vi "ni579x Load Characterization Data (EEPROM).vi"(0 "Register Bus":refnum<class "ni579x Register Bus v1 Host.lvclass">=refnum, 1 "scope":string(combo)="characterization data eeprom", 5 "start address":u32 format="%x", 7 "EEPROM Data Section":T1, 11 "Error In":errorcluster) -> (3 "EEPROM Header":T7 {"Product Code" format="%x"; "Checksum" format="%x"}, 4 "Register Bus (out)":refnum<class "ni579x Register Bus v1 Host.lvclass">, 6 "EEPROM Calibration Header":T6={"Checksum"=0, "Date"=timestamp(0 s since 1904-01-01), "Temperature"=0.0, "Misc. Info"="", "Pointer to Device Data Header"=0, "Number of Reserved Bytes"=28} {"Checksum" format="%x"}, 8 "Device Data Header":T5={"Checksum"=0, "Number of Channels"=0, "Number of Attenuations"=[], "Number of Attenuator Settings"=[], "Number of Gain Settings"=[], "Pointer to Cal Data"=[], "Number of Reserved Bytes"=7, "Number of Frequencies"=[]} {"Checksum" format="%x"}, 10 "Characterization Data":T2[](array[typedef]) {"Frequencies [Hz]" format="%#_6p"}, 15 "Error Out":errorcluster)   [LabVIEW 2013]
doc: "Reads characterization data from the on-device EEPROM and returns headers and an array of characterization data for each channel.\n\n<B>Input Parameters</B>\n\n<B>Register Bus</B> The Register Bus object created by the ni579x Open VI and used as the session handle for the NI-579x Configuration Design Library.\n\n<B>scope</B> The EEPROM to read characterization data from. The only option is \"characterization data eeprom\".\n\n<B>start address</B> The start offset of the data in the EEPROM.\n\n<B>EEPROM Data Section</B> The EEPROM can contain characterization data measured and calculated by the manufacturer (the Factory Data) as well as data measured and calculated by the user (the User Data).\n\n<B>Output Parameters</B>\n\n<B>Register Bus (out)</B> The Register Bus object created by the ni579x Open VI and used as the session handle for the NI-579x Configuration Design Library.\n\n<B>EEPROM Header</B> Header information for the entire EEPROM.\n\n<B>EEPROM Calibration Header</B> Header information describing the calibration sections.\n\n<B>Device Data Header</B> Header information describing the device characterization data sections.\n\n<B>Characterization Data</B> An array of characterization data for each channel.\nFor the 5791,\n the Rx channel is index 0\n the Tx channel is index 1\nFor the 5792,\n the Rx channel is index 0\nFor the 5793,\n the Tx channel is index 1"
uses:
  <instrlib>/ni579x/Register Bus/v1/Host/ni579x Register Bus v1 Host.lvclass
  <instrlib>/ni579x/Config/v1/Shared/Types/EEPROM/ni579x EEPROM Header.ctl
  <instrlib>/ni579x/Config/v1/Shared/Types/EEPROM/ni579x EEPROM Calibration Header.ctl
  <instrlib>/ni579x/Config/v1/Shared/Types/EEPROM/ni579x EEPROM Device Data Header.ctl
  <instrlib>/ni579x/Config/v1/Shared/Types/ni579x Characterization Data.ctl
  <instrlib>/ni579x/Config/v1/Shared/Types/ni579x IQ Imbalance.ctl
  <instrlib>/ni579x/Config/v1/Shared/Types/ni579x Gain to Attenuation Mapping.ctl
  <instrlib>/ni579x/Config/v1/Shared/Types/EEPROM/ni579x EEPROM Data Section.ctl
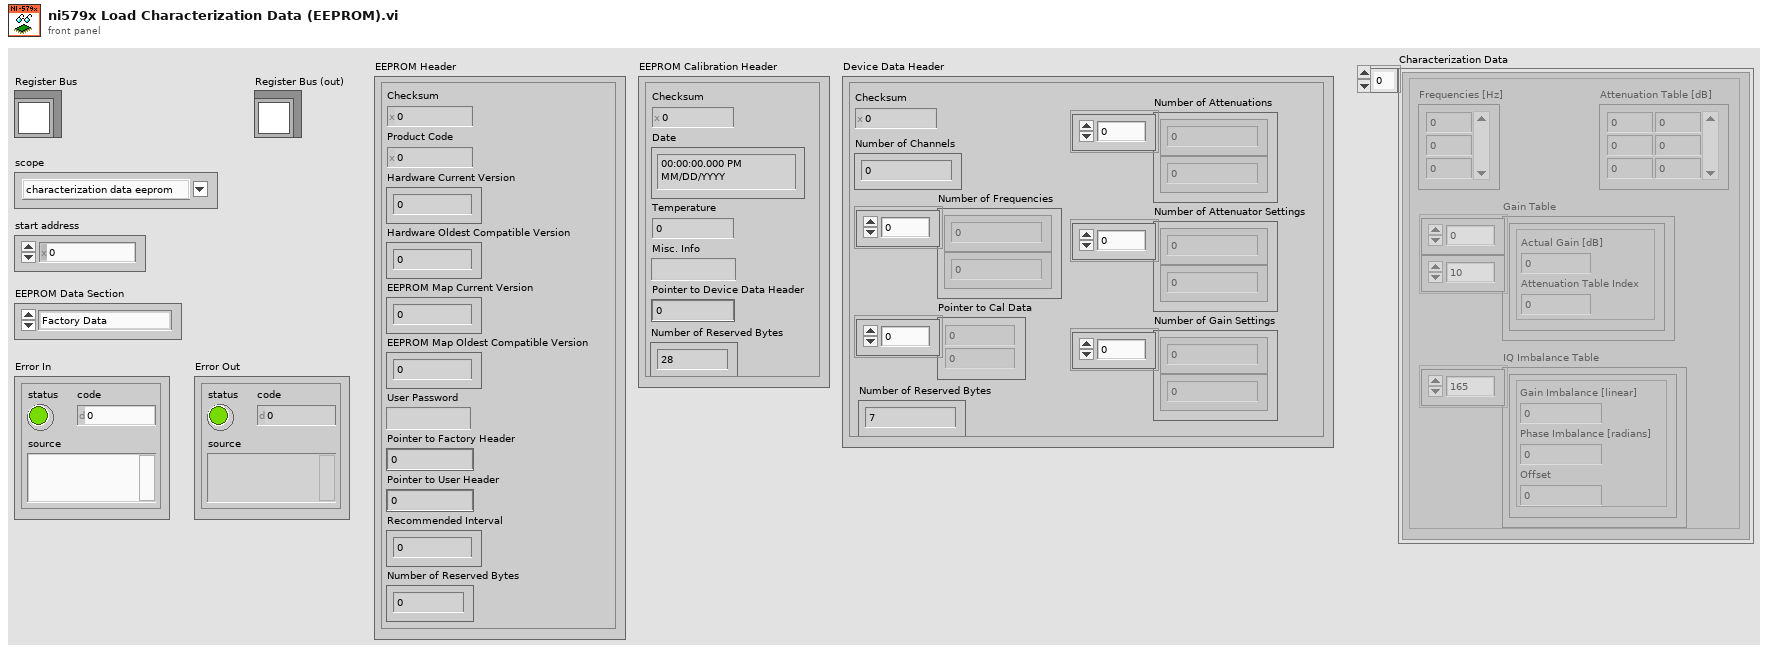
[diagram p1: front panel]
types:
  T1 = typedef "ni579x EEPROM Data Section.ctl" = enum16{"Factory Data", "User Data"}
  T2 = typedef "ni579x Characterization Data.ctl" = cluster{"Attenuation Table [dB]":dbl[][], "Frequencies [Hz]":dbl[], "IQ Imbalance Table":T3[], "Gain Table":T4[][]}
  T3 = typedef "ni579x IQ Imbalance.ctl" = cluster{"Gain Imbalance [linear]":dbl, "Phase Imbalance [radians]":dbl, "Offset":cdb}
  T4 = typedef "ni579x Gain to Attenuation Mapping.ctl" = cluster{"Actual Gain [dB]":dbl, "Attenuation Table Index":i32}
  T5 = typedef "ni579x EEPROM Device Data Header.ctl" = cluster{"Checksum":u32, "Number of Channels":u8, "Number of Attenuations":u16[], "Number of Attenuator Settings":u8[], "Number of Gain Settings":u8[], "Pointer to Cal Data":u32[], "Number of Reserved Bytes":i32, "Number of Frequencies":u16[]}
  T6 = typedef "ni579x EEPROM Calibration Header.ctl" = cluster{"Checksum":u32, "Date":timestamp, "Temperature":sgl, "Misc. Info":string, "Pointer to Device Data Header":u32, "Number of Reserved Bytes":i32}
  T7 = typedef "ni579x EEPROM Header.ctl" = cluster{"Checksum":u32, "Product Code":u16, "Hardware Current Version":u16, "Hardware Oldest Compatible Version":u16, "EEPROM Map Current Version":u16, "EEPROM Map Oldest Compatible Version":u16, "User Password":string, "Pointer to Factory Header":u32, "Pointer to User Header":u32, "Recommended Interval":u16, "Number of Reserved Bytes":i32}
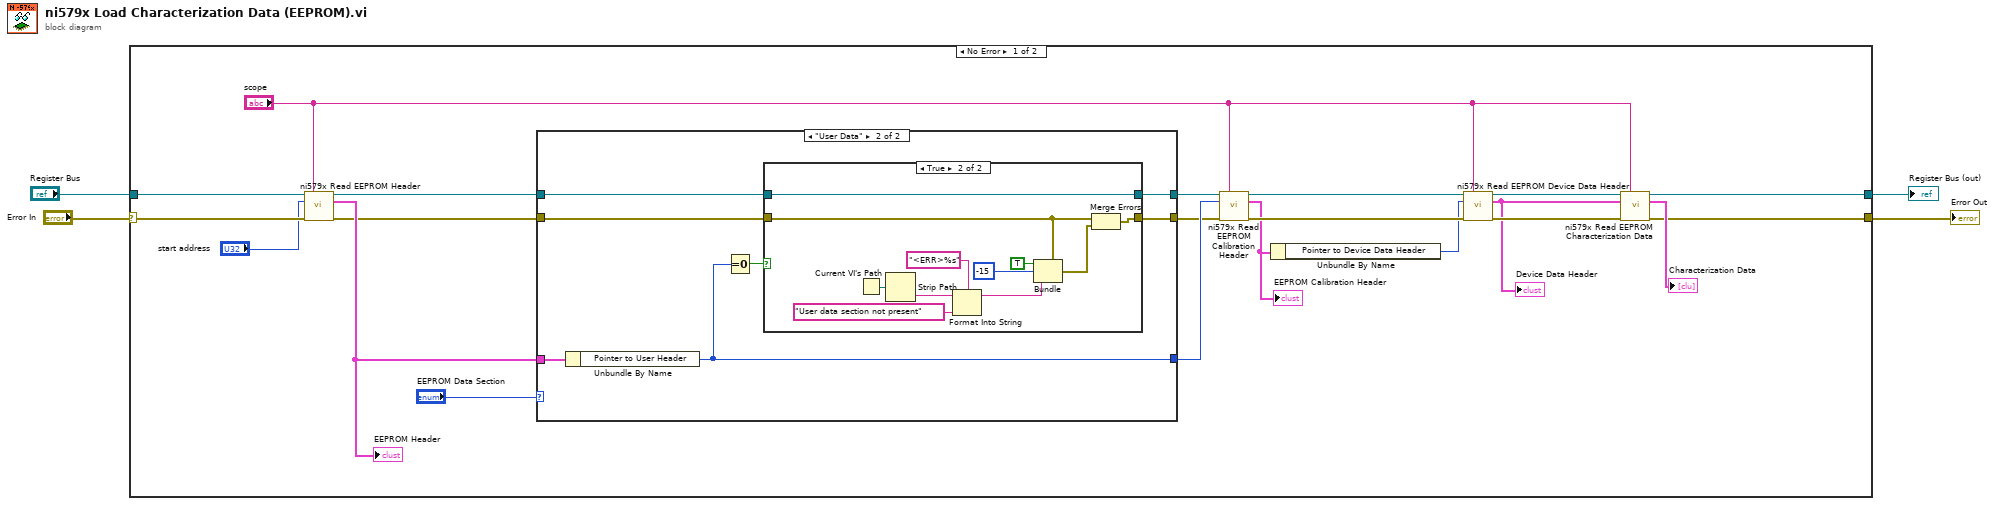
[diagram p0: block diagram]
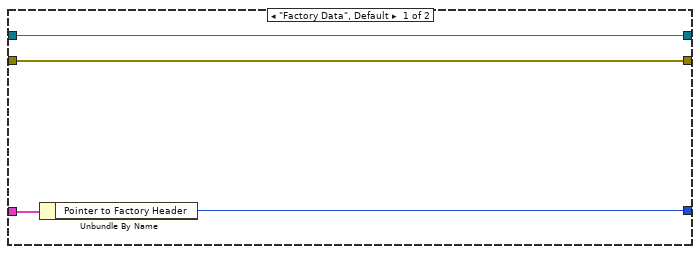
[diagram p2: hidden frame]
diagram:
  n1 = case shown="No Error" "Error In" {
    selector: "Error In" -> [w24 w51]
    tunnel: [w11 w51] -> w3
    tunnel: "Register Bus" -> [w25 w50]
    tunnel: [w12 w50] -> w1
    frame No Error {
      n2 = call <instrlib>:"ni579x Read EEPROM Header.vi"("Register Bus"=w25, "scope"="scope", "start address"="start address", "Error In"=w24) -> ("Register Bus (out)"=w8:refnum<class "ni579x Register Bus v1 Host.lvclass">, "EEPROM Header"=w13:T7, "Error Out"=w7:errorcluster)  [unwired: 9 in]
      "EEPROM Header" <- w13
      n3 = case shown="\"User Data\"" "EEPROM Data Section" {
        tunnel: [w29 w33] -> w14
        tunnel: w13 -> [w28 w36]
        tunnel: w8 -> [w27 w31]
        tunnel: w7 -> [w26 w35]
        tunnel: [w26 w34] -> w6
        tunnel: [w27 w30] -> w5
        frame "Factory Data", Default {
          n4 = Unbundle By Name(w28) -> ("Pointer to Factory Header"=w29:u32)
        }
        frame "User Data" {
          n5 = Unbundle By Name(w36) -> ("Pointer to User Header"=w33:u32)
          n6 = Equal To 0?(x=w33) -> (x = 0?=w32:bool)
          n7 = case shown="True" w32 {
            tunnel: w35 -> [w38 w41]
            tunnel: [w38 w40] -> w34
            tunnel: w31 -> [w37 w39]
            tunnel: [w37 w39] -> w30
            frame False {
            }
            frame True {
              n8 = Current VI's Path() -> (path=w48:path)
              n9 = Strip Path(path=w48) -> (name=w47:string)  [unwired: 1 out]
              n10 = Format Into String(format string="<ERR>%s", initial string=w47, "User data section not present" ("input 1")) -> (resulting string=w46:string)  [unwired: 1 in, 1 out]
              n11 = Bundle(cluster=w41, "status"=TRUE, "code"=-15, "source"=w46) -> (w45:errorcluster)
              n12 = Merge Errors(w41, w45) -> (w40:errorcluster)
            }
          }
        }
      }
      n13 = call <instrlib>:"ni579x Read EEPROM Calibration Header.vi"("Register Bus"=w5, "scope"="scope", "start address"=w14, "Error In"=w6) -> ("Register Bus (out)"=w21:refnum<class "ni579x Register Bus v1 Host.lvclass">, "EEPROM Calibration Header"=w20:T6, "Error Out"=w22:errorcluster)  [unwired: 9 in]
      "EEPROM Calibration Header" <- w20
      n14 = Unbundle By Name(w20) -> ("Pointer to Device Data Header"=w19:u32)
      n15 = call <instrlib>:"ni579x Read EEPROM Device Data Header.vi"("Register Bus"=w21, "scope"="scope", "start address"=w19, "Error In"=w22) -> ("Register Bus (out)"=w18:refnum<class "ni579x Register Bus v1 Host.lvclass">, "Device Data Header"=w16:T5, "Error Out"=w17:errorcluster)  [unwired: 9 in]
      "Device Data Header" <- w16
      n16 = call <instrlib>:"ni579x Read EEPROM Characterization Data.vi"("Register Bus"=w18, "scope"="scope", "Device Data Header"=w16, "Error In"=w17) -> ("Register Bus (out)"=w12:refnum<class "ni579x Register Bus v1 Host.lvclass">, "Characterization Data"=→"Characterization Data":T2[], "Error Out"=w11:errorcluster)  [unwired: 9 in]
    }
    frame Error {
    }
  }
  "Register Bus (out)" <- w1
  "Error Out" <- w3
